vi "Receive Value Change Event.vi"(8 "error in (no error)":errorcluster, 10 "ValueChangeMsg":refnum<class "ValueChangeMsg.lvclass">, 11 "OneButtonDialogBox In":refnum<class "TwoButtonDialogBox.lvclass">) -> (0 "error out":errorcluster, 3 "OneButtonDialogBox Out":refnum<class "TwoButtonDialogBox.lvclass">)   [LabVIEW 2020, in "TwoButtonDialogBox.lvlib" / "TwoButtonDialogBox.lvclass"]
doc: "<License>\nCopyright © 2017 Composed Systems, LLC | All rights reserved\nwww.composed.io\n\nAuthor: Ethan Stern <ethan.stern@composed.io>\n\nThis software is provided \"AS IS\" WITHOUT WARRANTIES, either express or implied, AND IS FOR EDUCATIONAL PURPOSES ONLY.\n</License>"
uses:
  <vilib>/gpm_packages/@cs/mva-dialogbox/source/TwoButtonDialobBox/TwoButtonDialogBox.lvclass
  C:/Program Files/National Instruments/LabVIEW 2020/vi.lib/ActorFramework/Actor/Actor.lvclass
  <vilib>/gpm_packages/@cs/mva-viewable/Source/ActorEvents/IEventAggregator Messages/ValueChangeMsg/ValueChangeMsg.lvclass
  <vilib>/gpm_packages/@cs/mva-viewable/Source/ActorEvents/IEventAggregator Messages/ValueChangeMsg/ValueChangeMsg.lvclass/ValueChangeMsg.ctl
  <vilib>/gpm_packages/@cs/mva-dialogbox/source/TwoButtonDialobBox/TwoButtonDialogBox.lvclass/TwoButtonDialogBox.ctl
  <vilib>/ActorFramework/Actor/Actor.lvclass/Actor.ctl
  <vilib>/ActorFramework/Message Enqueuer/Message Enqueuer.lvclass/Message Enqueuer.ctl
  <vilib>/gpm_packages/@cs/actor-framework-messages/Source/RoundTripMessage/RoundTripMessage.lvclass/RoundTripMessage.ctl
  <vilib>/ActorFramework/Message Enqueuer/Init from Existing Queue.vi
  <vilib>/ActorFramework/Message Enqueuer/Enqueue.vi
  <vilib>/gpm_packages/@cs/mva-dialogbox/source/IDialogBox/IDialogBox Messages/Dialog Return Msg/Dialog Return Msg.lvclass
  C:/Program Files/National Instruments/LabVIEW 2020/vi.lib/gpm_packages/@cs/actor-framework-messages/Source/RoundTripMessage/RoundTripMessage.lvclass
  <vilib>/gpm_packages/@cs/actor-framework-messages/Source/RoundTripMessage/RoundTripMessage.lvclass
  C:/Program Files/National Instruments/LabVIEW 2020/vi.lib/ActorFramework/Message/Message.lvclass
  <vilib>/ActorFramework/Stop Msg/Stop Msg.lvclass
  <vilib>/ActorFramework/Message Priority Queue/Priority Enqueue.vi
  <vilib>/ActorFramework/Message Enqueuer/Message Enqueuer.lvclass
  <vilib>/ActorFramework/Actor/Actor.lvclass
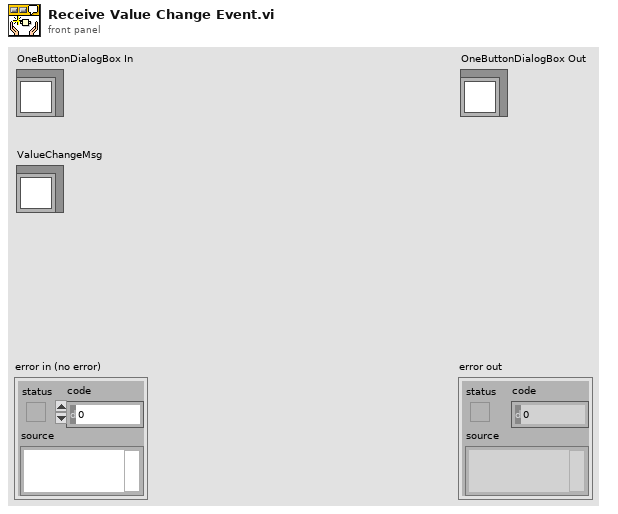
[diagram p1: front panel]
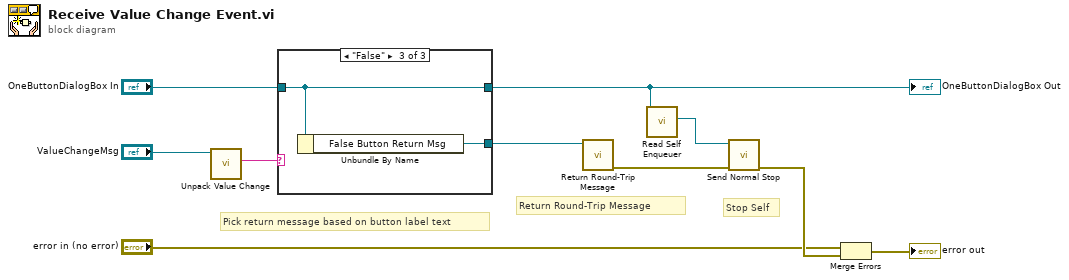
[diagram p0: block diagram]
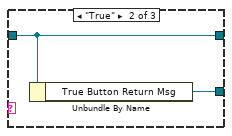
[diagram p3: hidden frame]
diagram:
  # "Pick return message based on button label text"
  # "Stop Self"
  # "Return Round-Trip Message"
  n1 = call <vilib>:"Unpack Value Change.vi"("ValueChangeMsg"="ValueChangeMsg") -> ("Control Label"=w1:string)  [unwired: 6 in, 4 out]
  n2 = case shown="\"False\"" w1 {
    tunnel: [_ w13 w15] -> w9
    tunnel: "OneButtonDialogBox In" -> [w11 w12 w14]
    tunnel: [w11 w12 w14] -> w2
    frame Default {
    }
    frame "True" {
      n3 = Unbundle By Name(w12) -> ("True Button Return Msg"=w13:refnum<class "Dialog Return Msg.lvclass">)
    }
    frame "False" {
      n4 = Unbundle By Name(w14) -> ("False Button Return Msg"=w15:refnum<class "Dialog Return Msg.lvclass">)
    }
  }
  "OneButtonDialogBox Out" <- w2
  n5 = call <vilib>:"Return Round-Trip Message.vi"("RoundTripMessage In"=w9) -> ("error out"=w8:errorcluster)  [unwired: 10 in]
  n6 = call <vilib>:"Read Self Enqueuer.vi"("Actor"=w2) -> ("Self Enqueuer"=w10:refnum<class "Message Enqueuer.lvclass">)  [unwired: 10 in]
  n7 = call <vilib>:"Send Normal Stop.vi"("error in (no error)"=w8, "Message Enqueuer"=w10) -> ("error out"=w7:errorcluster)  [unwired: 9 in]
  n8 = Merge Errors("error in (no error)", w7) -> (→"error out":errorcluster)
